vi "BOARDHDR_write.vi"(8 "error in (no error)":errorcluster, 10 "BOARDHDR":T1, 11 "refnum in":refnum<file>) -> (0 "error out":errorcluster, 3 "refnum out":refnum<file>)   [LabVIEW 2012]
uses:
  TTTR_data_headers/BOARDHDR.ctl
  TTTR_data_headers/RtChan.ctl
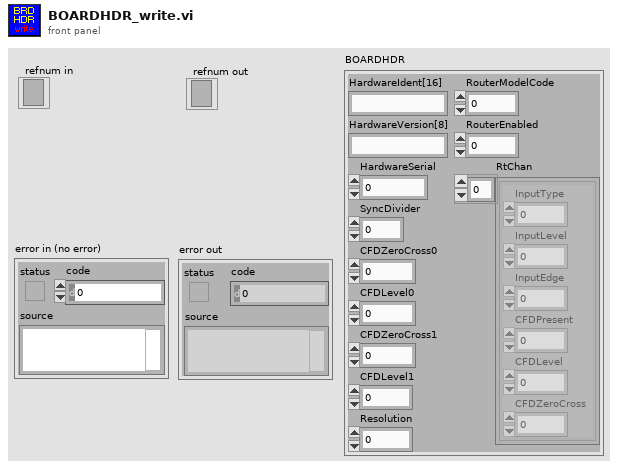
[diagram p1: front panel]
types:
  T1 = typedef "BOARDHDR.ctl" = cluster{"HardwareIdent[16]":string, "HardwareVersion[8]":string, "HardwareSerial":i32, "SyncDivider":i32, "CFDZeroCross0":i32, "CFDLevel0":i32, "CFDZeroCross1":i32, "CFDLevel1":i32, "Resolution":sgl, "RouterModelCode":i32, "RouterEnabled":i32, "RtChan":T2}
  T2 = typedef "RtChan.ctl" = cluster{"InputType":i32, "InputLevel":i32, "InputEdge":i32, "CFDPresent":i32, "CFDLevel":i32, "CFDZeroCross":i32}[]
  T3 = enum16{"big-endian, network order", "native, host order", "little-endian"}
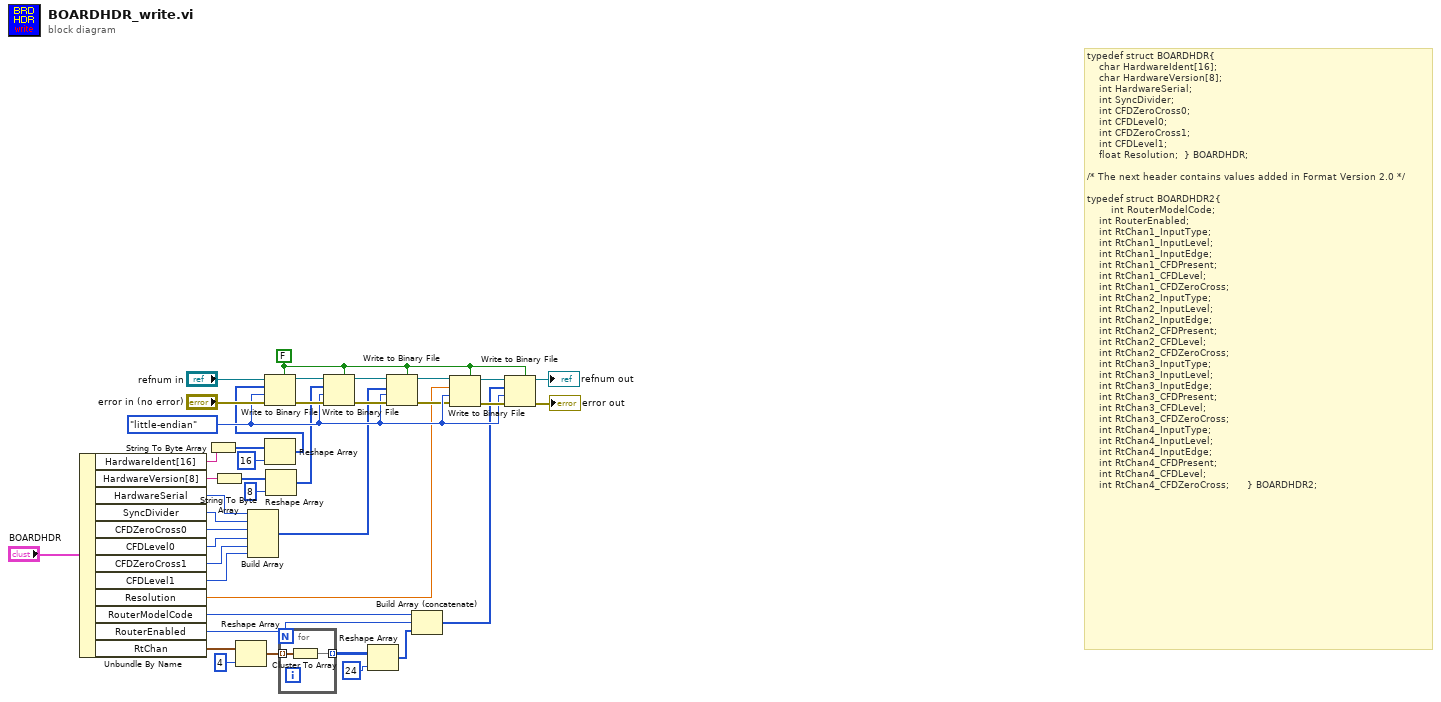
[diagram p0: block diagram]
diagram:
  w18 = FALSE ("prepend array or string size? (T)")
  w32 = T3."little-endian" ("byte order (0:big-endian, network order)")
  # "typedef struct BOARDHDR{\t\t\n\t\t\t\tchar HardwareIdent[16]; \n\t\t\t\tchar HardwareVersion[8]; \n\t\t\t\tint HardwareSerial; \n\t\t\t\tint SyncDivider;\n\t\t\t\tint CFDZeroCross0;\n\t\t\t\tint CFDLevel0;\n\t\t\t\tint CFDZeroCross1;\n\t\t\t\tint CFDLevel1;\n\t\t\t\tfloat Resolution;\t\t} BOARDHDR;\n\t\t\t\t\n/* The next header contains values added in Format Version 2.0 */\n\ntypedef struct BOARDHDR2{\n        int RouterModelCode;\n\t\t\t\tint RouterEnabled;\n\t\t\t\tint RtChan1_InputType; \n\t\t\t\tint RtChan1_InputLevel;\n\t\t\t\tint RtChan1_InputEdge;\n\t\t\t\tint RtChan1_CFDPresent;\n\t\t\t\tint RtChan1_CFDLevel;\n\t\t\t\tint RtChan1_CFDZeroCross;\n\t\t\t\tint RtChan2_InputType; \n\t\t\t\tint RtChan2_InputLevel;\n\t\t\t\tint RtChan2_InputEdge;\n\t\t\t\tint RtChan2_CFDPresent;\n\t\t\t\tint RtChan2_CFDLevel;\n\t\t\t\tint RtChan2_CFDZeroCross;\n\t\t\t\tint RtChan3_InputType; \n\t\t\t\tint RtChan3_InputLevel;\n\t\t\t\tint RtChan3_InputEdge;\n\t\t\t\tint RtChan3_CFDPresent;\n\t\t\t\tint RtChan3_CFDLevel;\n\t\t\t\tint RtChan3_CFDZeroCross;\n\t\t\t\tint RtChan4_InputType; \n\t\t\t\tint RtChan4_InputLevel;\n\t\t\t\tint RtChan4_InputEdge;\n\t\t\t\tint RtChan4_CFDPresent;\n\t\t\t\tint RtChan4_CFDLevel;\n\t\t\t\tint RtChan4_CFDZeroCross;      } BOARDHDR2;"
  n1 = Unbundle By Name("BOARDHDR") -> ("HardwareIdent[16]"=w26:string, "HardwareVersion[8]"=w25:string, "HardwareSerial"=w17:i32, "SyncDivider"=w16:i32, "CFDZeroCross0"=w15:i32, "CFDLevel0"=w14:i32, "CFDZeroCross1"=w13:i32, "CFDLevel1"=w12:i32, "Resolution"=w10:sgl, "RouterModelCode"=w4:i32, "RouterEnabled"=w3:i32, "RtChan"=w9:T2)
  n2 = String To Byte Array(string=w26) -> (unsigned byte array=w24:u8[])
  n3 = String To Byte Array(string=w25) -> (unsigned byte array=w20:u8[])
  n4 = Reshape Array(w9, 4 ("dimension size")) -> (w7:T2)
  n5 = Build Array(w17, w16, w15, w14, w13, w12) -> (w11:i32[])
  n6 = Reshape Array(w24, 16 ("dimension size")) -> (w22:u8[])
  n7 = Write to Binary File(file (use dialog)="refnum in", data=w22, error in="error in (no error)", 5:w18, 9:w32) -> (refnum out=w39:refnum<file>, error out=w40:errorcluster)  [unwired: 1 in, 1 out]
  n8 = Reshape Array(w20, 8 ("dimension size")) -> (w19:u8[])
  n9 = for {
    tunnel: w7 -> [w42] mode=indexing
    tunnel: [w41] -> w6 mode=indexing
    n10 = Cluster To Array(cluster=w42) -> (array=w41:i32[])
  }
  n11 = Write to Binary File(file (use dialog)=w39, data=w19, error in=w40, 5:w18, 9:w32) -> (refnum out=w37:refnum<file>, error out=w38:errorcluster)  [unwired: 1 in, 1 out]
  n12 = Reshape Array(w6, 24 ("dimension size")) -> (w2:i32[])
  n13 = Write to Binary File(file (use dialog)=w37, data=w11, error in=w38, 5:w18, 9:w32) -> (refnum out=w31:refnum<file>, error out=w30:errorcluster)  [unwired: 1 in, 1 out]
  n14 = Build Array (concatenate)(w4, w3, w2) -> (w1:i32[])
  n15 = Write to Binary File(file (use dialog)=w31, data=w10, error in=w30, 5:w18, 9:w32) -> (refnum out=w35:refnum<file>, error out=w36:errorcluster)  [unwired: 1 in, 1 out]
  n16 = Write to Binary File(file (use dialog)=w35, data=w1, error in=w36, 5:w18, 9:w32) -> (refnum out=→"refnum out":refnum<file>, error out=→"error out":errorcluster)  [unwired: 1 in, 1 out]
